vi "Read Joystick Input.vi"(1 "Input Array":dbl[](array[numeric])) -> (0 "Appended Array":dbl[](array[numeric]))   [LabVIEW 2014]
uses:
  Begin/Global Variables.vi
panel:
  out "Driver Joystick X2":dbl
  out "Driver Joystick Y1":dbl
  out "Driver Joystick X1":dbl
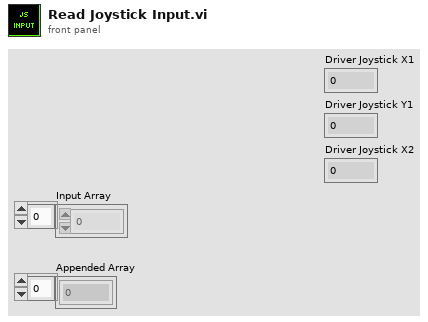
[diagram p1: front panel]
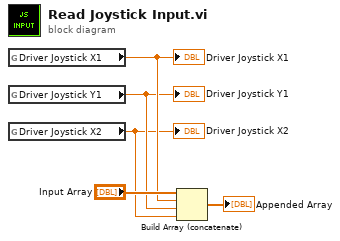
[diagram p0: block diagram]
diagram:
  n1 = global read "Global Variables.vi" "Driver Joystick X1"() -> (w4:dbl)
  "Driver Joystick X1" <- w4
  n2 = global read "Global Variables.vi" "Driver Joystick Y1"() -> (w3:dbl)
  "Driver Joystick Y1" <- w3
  n3 = global read "Global Variables.vi" "Driver Joystick X2"() -> (w2:dbl)
  "Driver Joystick X2" <- w2
  n4 = Build Array (concatenate)("Input Array", w4, w3, w2) -> (→"Appended Array":dbl[])
